vi "mqtt_subsriber.vi"() -> ()   [LabVIEW 2024]
uses:
  <vilib>/LabVIEW Open Source Project/MQTT Control Packets/Control Packets/SUBSCRIBE/Topic Subscription -- cluster.ctl
  <vilib>/LabVIEW Open Source Project/MQTT Control Packets/Control Packets/ControlPacket/QualityOfService -- enum.ctl
  <vilib>/LabVIEW Open Source Project/MQTT Client/Client class/Client.lvclass/Client.ctl
  <vilib>/LabVIEW Open Source Project/Connection/Connection.TCP/Connection.TCP.lvclass
  C:/Program Files (x86)/National Instruments/LabVIEW 2024/vi.lib/LabVIEW Open Source Project/Connection/Connection/Connection.lvclass
  <vilib>/LabVIEW Open Source Project/MQTT Client/Client class/Client.lvclass
  C:/Program Files (x86)/National Instruments/LabVIEW 2024/vi.lib/LabVIEW Open Source Project/MQTT Connection/MQTT_Base/Base Class/MQTT_Base.lvclass
  <vilib>/LabVIEW Open Source Project/MQTT Control Packets/Control Packets/PUBLISH/PUBLISH.lvclass
  <vilib>/LabVIEW Open Source Project/MQTT Connection/MQTT_Base/Base Class/MQTT_Base.lvclass
  <vilib>/LabVIEW Open Source Project/MQTT Control Packets/Control Packets/ControlPacket/ControlPacket.lvclass
  <vilib>/LabVIEW Open Source Project/MQTT Control Packets/Control Packets/SUBSCRIBE/SUBSCRIBE.lvclass
panel:
  out "String 2":string
  out "String":string
  out "Numeric 3":sgl format="%.3f"
  out "Numeric 2":sgl format="%.5f"
  out "Numeric":i32
  in  "stop":bool
  out "connected":bool
  out "last error":errorcluster
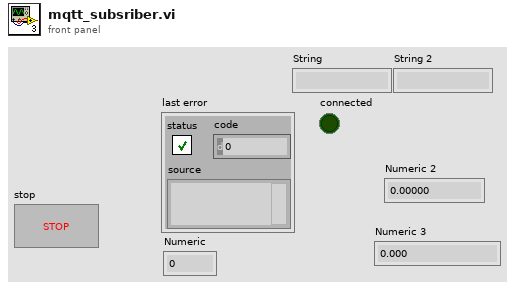
[diagram p1: front panel]
types:
  T1 = typedef "MQTT_Control_Packets.lvlib/SUBSCRIBE.lvclass/Topic Subscription -- cluster.ctl" = cluster{"Topic Filter":string, "QoS":T2}
  T2 = typedef "MQTT_Control_Packets.lvlib/ControlPacket.lvclass/QualityOfService -- enum.ctl" = enum16{"0 (At Most Once)", "1 (At Least Once)", "2 (Exactly Once)"}
  T3 = typedef "MQTT Client.lvlib/Client.lvclass/Public Events -- cluster.ctl" = cluster{"Connection Status":refnum<user-event>, "Connected":refnum<user-event>, "Application Message":refnum<user-event>}
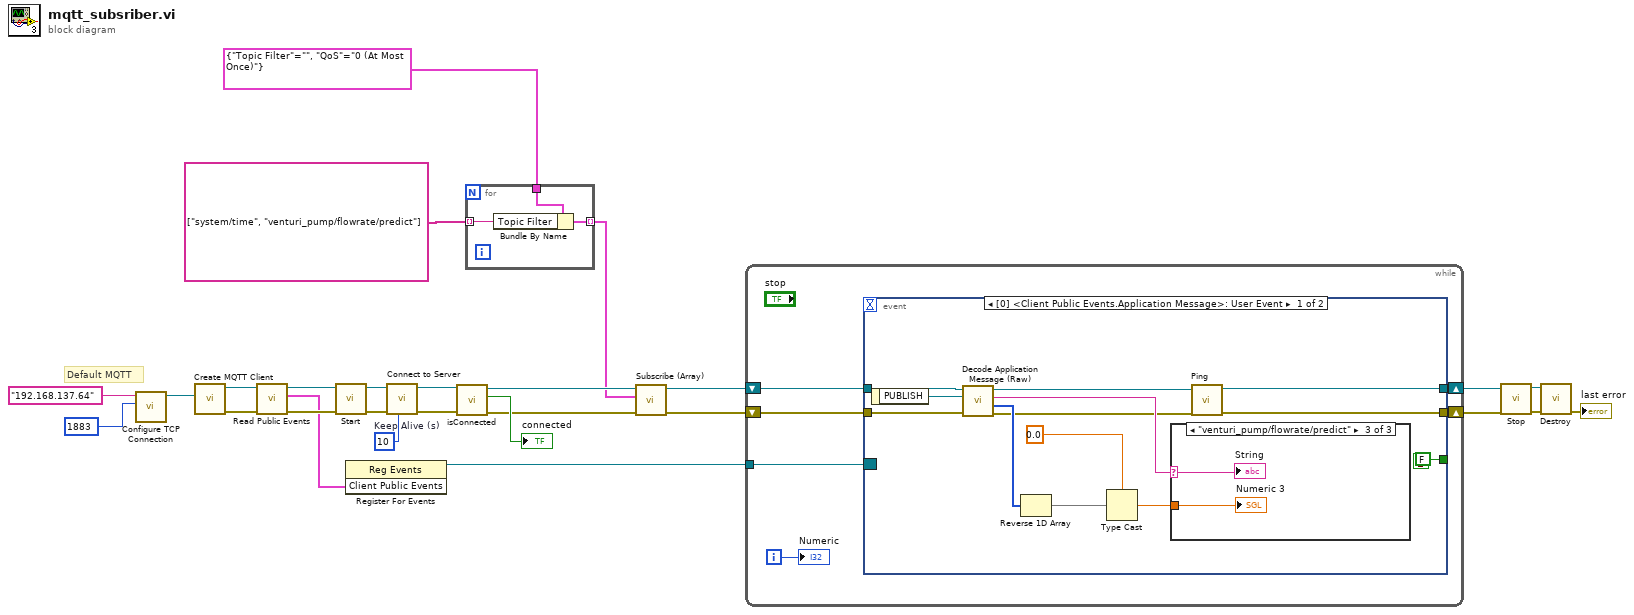
[diagram p0: block diagram]
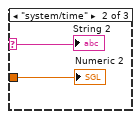
[diagram p3: hidden frame]
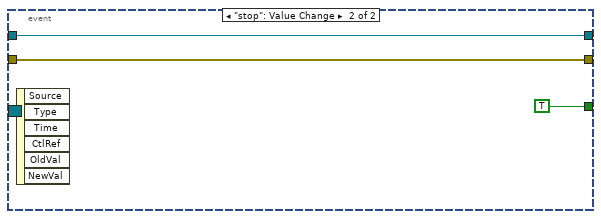
[diagram p4: hidden frame]
diagram:
  w8 = u16 10  # Keep Alive (s)
  # "Default MQTT"
  n1 = call <vilib>:"Configure TCP Connection.vi"("remote port (80)"=u16 1883, "address (localhost)"="192.168.137.64") -> ("Connection.TCP"=w27:refnum<class "Connection.TCP.lvclass">)  [unwired: 8 in, 1 out]
  n2 = call <vilib>:"Create MQTT Client.vi"("Connection Configuration"=w27) -> ("error out"=w13:errorcluster, "Client out"=w14:refnum<class "Client.lvclass">)  [unwired: 9 in]
  n3 = call <vilib>:"Read Public Events.vi"("error in (no error)"=w13, "Client in"=w14) -> ("error out"=w11:errorcluster, "Client Public Events"=w10:T3, "Client out"=w12:refnum<class "Client.lvclass">)  [unwired: 7 in]
  n4 = call <vilib>:"Start.vi"("error in (no error)"=w11, "MQTT_Base in"=w12) -> ("error out"=w17:errorcluster, "MQTT_Base out"=w18:refnum<class "Client.lvclass">)  [unwired: 7 in, 1 out]
  n5 = register-events(w10) -> (reference out=w9:refnum<event-registration>)  [unwired: 2 in, 1 out]
  n6 = call <vilib>:"Connect to Server.vi"("Keep Alive (s)"=w8, "error in (no error)"=w17, "Client in"=w18) -> ("error out"=w15:errorcluster, "Client out"=w16:refnum<class "Client.lvclass">)  [unwired: 5 in, 2 out]
  n7 = call <vilib>:"isConnected.vi"("error in (no error)"=w15, "Client in"=w16) -> ("error out"=w6:errorcluster, "connected"=→"connected":bool, "Client out"=w7:refnum<class "Client.lvclass">)  [unwired: 7 in]
  n8 = for {
    tunnel: string[] ["system/time", "venturi_pump/flowrate/predict"] -> [w30] mode=indexing
    tunnel: T1 {"Topic Filter"="", "QoS"=enum."0 (At Most Once)"} ("Topic Subscription") -> [w29]
    tunnel: [w28] -> w2 mode=indexing
    n9 = Bundle By Name(cluster=w29, "Topic Filter"=w30) -> (w28:T1)
  }
  n10 = call <vilib>:"Subscribe (Array).vi"("error in (no error)"=w6, "Topic Subscriptions"=w2, "Client in"=w7) -> ("error out"=w5:errorcluster, "Client out"=w4:refnum<class "Client.lvclass">)  [unwired: 6 in, 1 out]
  n11 = while {
    shift-right: [w35] -> w21
    shift-left: w4 -> [w37]
    shift-right: [w34] -> w20
    shift-left: w5 -> [w36]
    tunnel: w9 -> [w33]
    i -> [w32]
    stop <- w31 stop-if-true
    n12 = event shown="[0] <Client Public Events.Application Message>: User Event" {
      selector: w33 -> [_ _]
      dyn-events: _ -> [_ _]
      timeout: _ -> [_ _]
      tunnel: w37 -> [w49 w56]
      tunnel: w36 -> [w48 w55]
      tunnel: [w39 w56] -> w35
      tunnel: [w38 w55] -> w34
      tunnel: [FALSE TRUE] -> w31
      event User Event {
        n13 = event-data() -> ("PUBLISH"=w46:refnum<class "PUBLISH.lvclass">)  [unwired: 1 in]
        n14 = call <vilib>:"Decode Application Message (Raw).vi"("error in (no error)"=w48, "PUBLISH"=w46, "Client in"=w49) -> ("error out"=w40:errorcluster, "Payload"=w47:u8[], "Topic"=w43:string, "Client out"=w41:refnum<class "Client.lvclass">)  [unwired: 5 in]
        n15 = Reverse 1D Array(array=w47) -> (reversed array=w45:u8[])
        n16 = Type Cast(type=sgl 0.0, x=w45) -> (*(type *) &x=w42:sgl)
        n17 = case shown="\"venturi_pump/flowrate/predict\"" w43 {
          selector: w43 -> [_ w51 w53]
          tunnel: w42 -> [_ w52 w54]
          frame "False", Default {
          }
          frame "system/time" {
            "Numeric 2" <- w52
            "String 2" <- w51
          }
          frame "venturi_pump/flowrate/predict" {
            "Numeric 3" <- w54
            "String" <- w53
          }
        }
        n18 = call <vilib>:"Ping.vi"("error in (no error)"=w40, "Client in"=w41) -> ("error out"=w38:errorcluster, "Client out"=w39:refnum<class "Client.lvclass">)  [unwired: 6 in, 2 out]
      }
      event "stop": Value Change {
        n19 = event-data() -> ()  [unwired: 1 in, 6 out]
      }
    }
    "Numeric" <- w32
  }
  n20 = call <vilib>:"Stop.vi"("error in (no error)"=w20, "MQTT_Base in"=w21) -> ("error out"=w25:errorcluster, "MQTT_Base out"=w24:refnum<class "Client.lvclass">)  [unwired: 7 in, 1 out]
  n21 = call <vilib>:"Destroy.vi"("error in (no error)"=w25, "MQTT_Base in"=w24) -> ("error out"=→"last error":errorcluster)  [unwired: 8 in, 1 out]
